vi "24_Read and Write using File.vi"() -> ()   [LabVIEW 2022 SP3]
panel:
  in  "OK Button":bool
  in  "stop":bool
  out "Text read from file":string
  in  "Text to be written":string
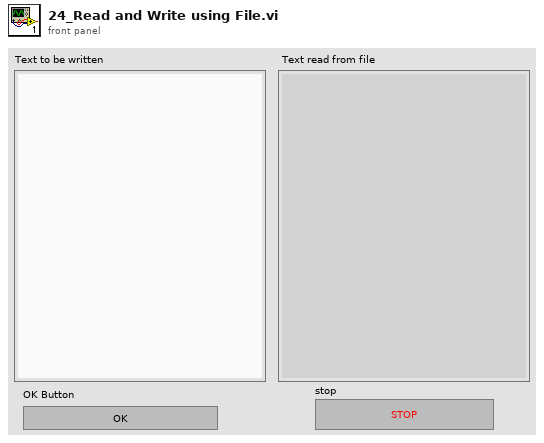
[diagram p1: front panel]
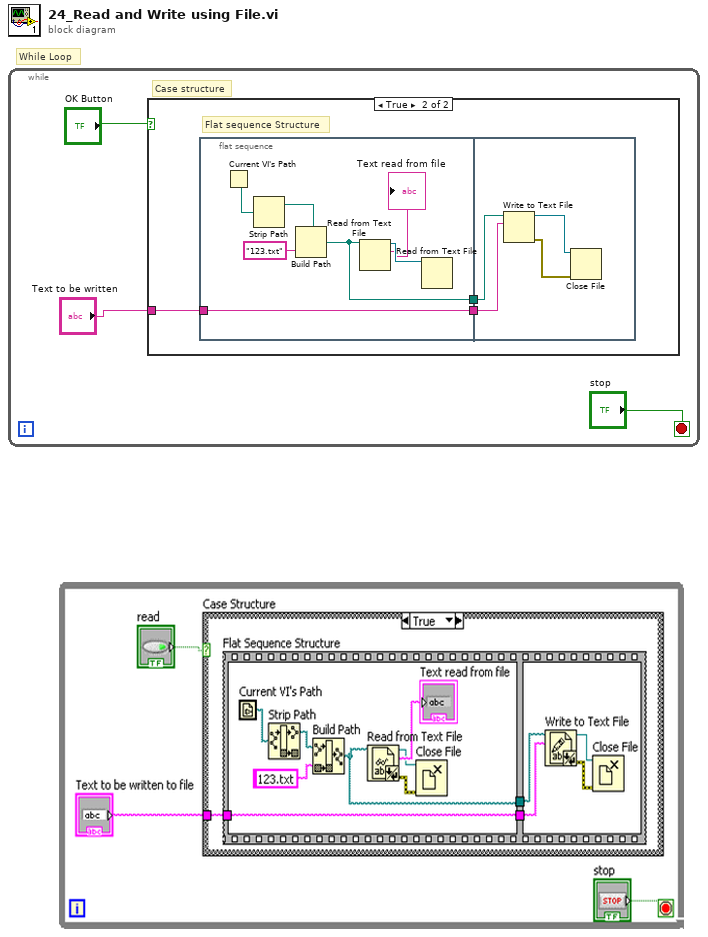
[diagram p0: block diagram]
diagram:
  # "While Loop"
  n1 = while {
    stop <- "stop" stop-if-true
    # "Case structure"
    n2 = case shown="True" "OK Button" {
      tunnel: "Text to be written" -> [_ w4]
      frame False {
      }
      frame True {
        # "Flat sequence Structure"
        n3 = flat-sequence {
          tunnel: [w11] -> w6
          tunnel: [w10] -> w5
          tunnel: w4 -> [w10]
          tunnel: w6 -> [w17]
          tunnel: w5 -> [w16]
          frame #0 {
            n4 = Current VI's Path() -> (path=w8:path)
            n5 = Strip Path(path=w8) -> (stripped path=w13:path)  [unwired: 1 out]
            n6 = Build Path(base path=w13, name or relative path="123.txt") -> (appended path=w11:path)
            n7 = Read from Text File(file (use dialog)=w11) -> (refnum out=w12:refnum<file>, text=→"Text read from file":string)  [unwired: 3 in, 2 out]
            n8 = Read from Text File(file (use dialog)=w12) -> ()  [unwired: 3 in, 4 out]
          }
          frame #1 {
            n9 = Write to Text File(file (use dialog)=w17, text=w16) -> (refnum out=w14:refnum<file>, error out=w15:errorcluster)  [unwired: 2 in, 1 out]
            n10 = Close File(refnum=w14, error in=w15) -> ()  [unwired: 2 out]
          }
        }
      }
    }
  }
